vi "Close Connections.vi"(8 "error in (no error)":errorcluster, 11 "CIF_UI in":refnum<class "CIF_UI.lvclass">) -> (0 "error out":errorcluster, 3 "CIF_UI out":refnum<class "CIF_UI.lvclass">)   [LabVIEW 2021, in "CIF_UI.lvclass"]
uses:
  CIF_UI.lvclass
  CIF_UI.lvclass/CIF_UI.ctl
  <vilib>/gRPC/LabVIEW gRPC Library/Shared/grpcId.ctl
  Typedef/Plugin Connection Map.ctl
  Typedef/Plugin Connections.ctl
  Typedef/PluginInfo.ctl
  Typedef/Version.ctl
  CIFCore/Common/Typedef/gRPC Reported Plugin Status.ctl
  CIFCore/Common/Typedef/Plugin State.ctl
  CIFCore/Common/Typedef/Timing Statistics.ctl
  CIFCore/Common/Typedef/Timing Stats Base.ctl
  CIFCore/Common/Typedef/FIFO Statistics.ctl
  CIFCore/Common/Typedef/Simple Error.ctl
  CIFCore/Common/Typedef/Monitor Doubles.ctl
  CIFCore/Common/Typedef/Monitor U64.ctl
  CIFCore/Common/Typedef/Monitor I64.ctl
  CIFPluginManager/CIFPluginManager/gRPC/CIF_Manager_Client_Wrapper/CIFManagerClientWrapper.lvlib
  <vilib>/gRPC/LabVIEW gRPC Library/grpc-lvsupport-release.lvlib
  CIFCore/Common/CIFCoreCommon.lvlib
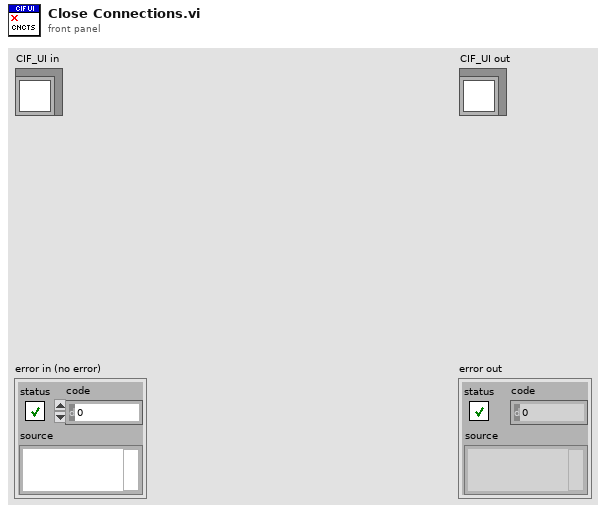
[diagram p1: front panel]
types:
  T1 = typedef "CIF_UI.lvclass/Plugin Connection Map.ctl" = map{string, T2}
  T2 = typedef "CIF_UI.lvclass/Plugin Connections.ctl" = cluster{"gRPC ID":T3, "Plugin Info":T4}
  T3 = typedef "grpc-lvsupport-release.lvlib/grpcId.ctl" = u64
  T4 = typedef "CIF_UI.lvclass/PluginInfo.ctl" = cluster{"Name":string, "Type":string, "grpc_port":i32, "Version":T5, "Node Status":T6}
  T5 = typedef "CIF_UI.lvclass/Version.ctl" = cluster{"Major":i32, "Minor":i32, "Fix":i32}
  T6 = typedef "CIFCoreCommon.lvlib/gRPC Reported Plugin Status.ctl" = cluster{"State":T7, "Timing Statistics (us)":T8, "FIFO Statistics (us)":T10, "error":T11, "Monitor Doubles":T12, "Monitor U64":T13, "Monitor I64":T14}
  T7 = typedef "CIFCoreCommon.lvlib/Plugin State.ctl" = enum32{"Null", "Creating", "Listening", "Running", "CleaningUp", "Destroying"}
  T8 = typedef "CIFCoreCommon.lvlib/Timing Statistics.ctl" = cluster{"Period":T9, "Wake Error":T9, "Execute":T9, "Housekeep":T9, "Idle":T9, "Cleanup":T9, "Custom 1 (custom units)":T9, "Custom 2 (custom units)":T9}
  T9 = typedef "CIFCoreCommon.lvlib/Timing Stats Base.ctl" = cluster{"Max":i64, "Avg":dbl, "Min":i64}
  T10 = typedef "CIFCoreCommon.lvlib/FIFO Statistics.ctl" = cluster{"From T0":T9, "From Previous Plugin":T9, "Output Error":T9}
  T11 = typedef "CIFCoreCommon.lvlib/Simple Error.ctl" = cluster{"status":bool, "code":i32}
  T12 = typedef "CIFCoreCommon.lvlib/Monitor Doubles.ctl" = cluster{"1":dbl, "2":dbl, "3":dbl, "4":dbl}
  T13 = typedef "CIFCoreCommon.lvlib/Monitor U64.ctl" = cluster{"1":u64, "2":u64, "3":u64, "4":u64}
  T14 = typedef "CIFCoreCommon.lvlib/Monitor I64.ctl" = cluster{"1":i64, "2":i64, "3":i64, "4":i64}
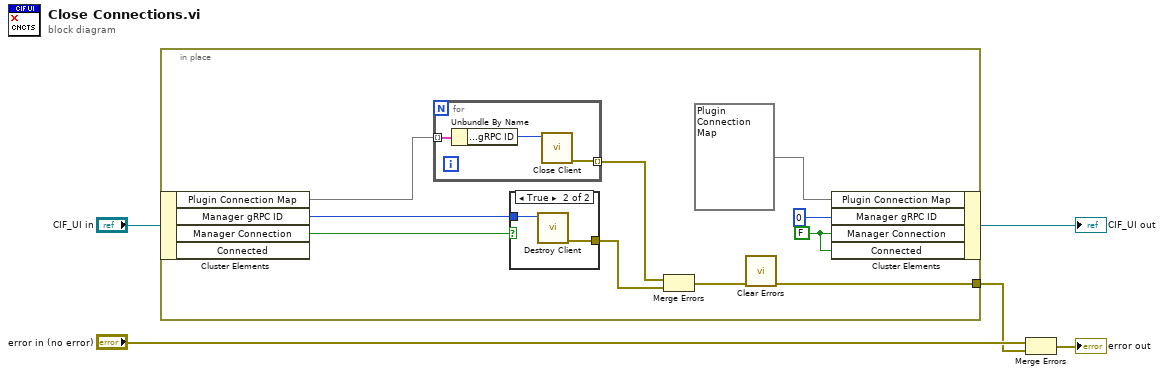
[diagram p0: block diagram]
diagram:
  n1 = in-place {
    in-place-border: [w6] -> w2
    w8 = FALSE ("Instrument Studio")
    n2 = in-place-cluster #1("CIF_UI in") -> ("Plugin Connection Map"=w13:T1, "Manager gRPC ID"=w15:T3, "Manager Connection"=w10:bool)  [unwired: 1 out]
    n3 = for {
      tunnel: w13 -> [w18] mode=indexing
      tunnel: [w16] -> w12 mode=indexing
      n4 = Unbundle By Name(w18) -> ("Plugin Connections.gRPC ID"=w17:T3)
      n5 = call <vilib>:"Close Client.vi"("ClientID in"=w17) -> ("error out"=w16:errorcluster)  [unwired: 10 in]
    }
    n6 = case shown="True" w10 {
      tunnel: w15 -> [_ w20]
      tunnel: [_ w19] -> w9
      frame False {
      }
      frame True {
        n7 = call "Destroy Client.vi"("gRPC ID"=w20) -> ("error out"=w19:errorcluster)  [unwired: 10 in]
      }
    }
    n8 = Merge Errors(w12, w9) -> (w7:errorcluster)
    n9 = call <vilib>:"Clear Errors.vi"("error in (no error)"=w7) -> ("error out"=w6:errorcluster)  [unwired: 5 in, 1 out]
    n10 = in-place-cluster #1("Plugin Connection Map"=T1 {}, "Manager gRPC ID"=T3 0 ("gRPC ID"), "Manager Connection"=w8, "Connected"=w8) -> (→"CIF_UI out":refnum<class "CIF_UI.lvclass">)
  }
  n11 = Merge Errors("error in (no error)", w2) -> (→"error out":errorcluster)
